vi "Main Target.vi"   [LabVIEW 2018]
uses:
  <vilib>/Platform/TimedLoop/XDataNode/timing_clust.ctl
  <vilib>/Platform/TimedLoop/XDataNode/nitl_modes.ctl
  <vilib>/Platform/TimedLoop/XDataNode/wakeup.ctl
  Host Messages.ctl
  Target Logging Cluster.ctl
  Target Sensors.ctl
  <vilib>/platform/TimedLoop/XDataNode/XDataNode.xnode
  <vilib>/Platform/TimedLoop/XDataNode/XDNodeRunTimeDep.lvlib
types:
  T1 = typedef "XDNodeRunTimeDep.lvlib/timing_clust.ctl" = cluster{"Expected End [f-1]":u64, "Actual End [f-1]":u64, "Finished Late? [f-1]":bool, "Expected End [i-1]":u64, "Actual End [i-1]":u64, "Finished Late? [i-1]":bool, "Expected Start [i]":u64, "Actual Start [i]":u64, "Expected Start [f]":u64, "Actual Start [f]":u64, "Source Name":string, "Structure Name":string, "Period":i64, "Deadline":i64, "Offset":i64, "Start":i64, "Priority":i32, "Timeout":i32, "Mode":T2, "Wakeup Reason":T3, "Error":errorcluster, "Source Type":string, "Secondary Source Type":string, "Global End Time":u64, "Global Start Time":u64, "Frame Duration":u64, "Iteration Duration":u64, "Assigned CPU":i32, "I/O Scan Engine Mode":u32}
  T2 = typedef "XDNodeRunTimeDep.lvlib/nitl_modes.ctl" = enum32{"No Change", "Process missed periods, maintain original phase", "Discard missed periods, maintain original phase", "Process missed periods, ignore original phase", "Discard missed periods, ignore original phase"}
  T3 = typedef "XDNodeRunTimeDep.lvlib/wakeup.ctl" = enum32{"Normal", "Aborted", "Asynchronous wakeup", "Timing source error", "Timed loop error", "Timeout"}
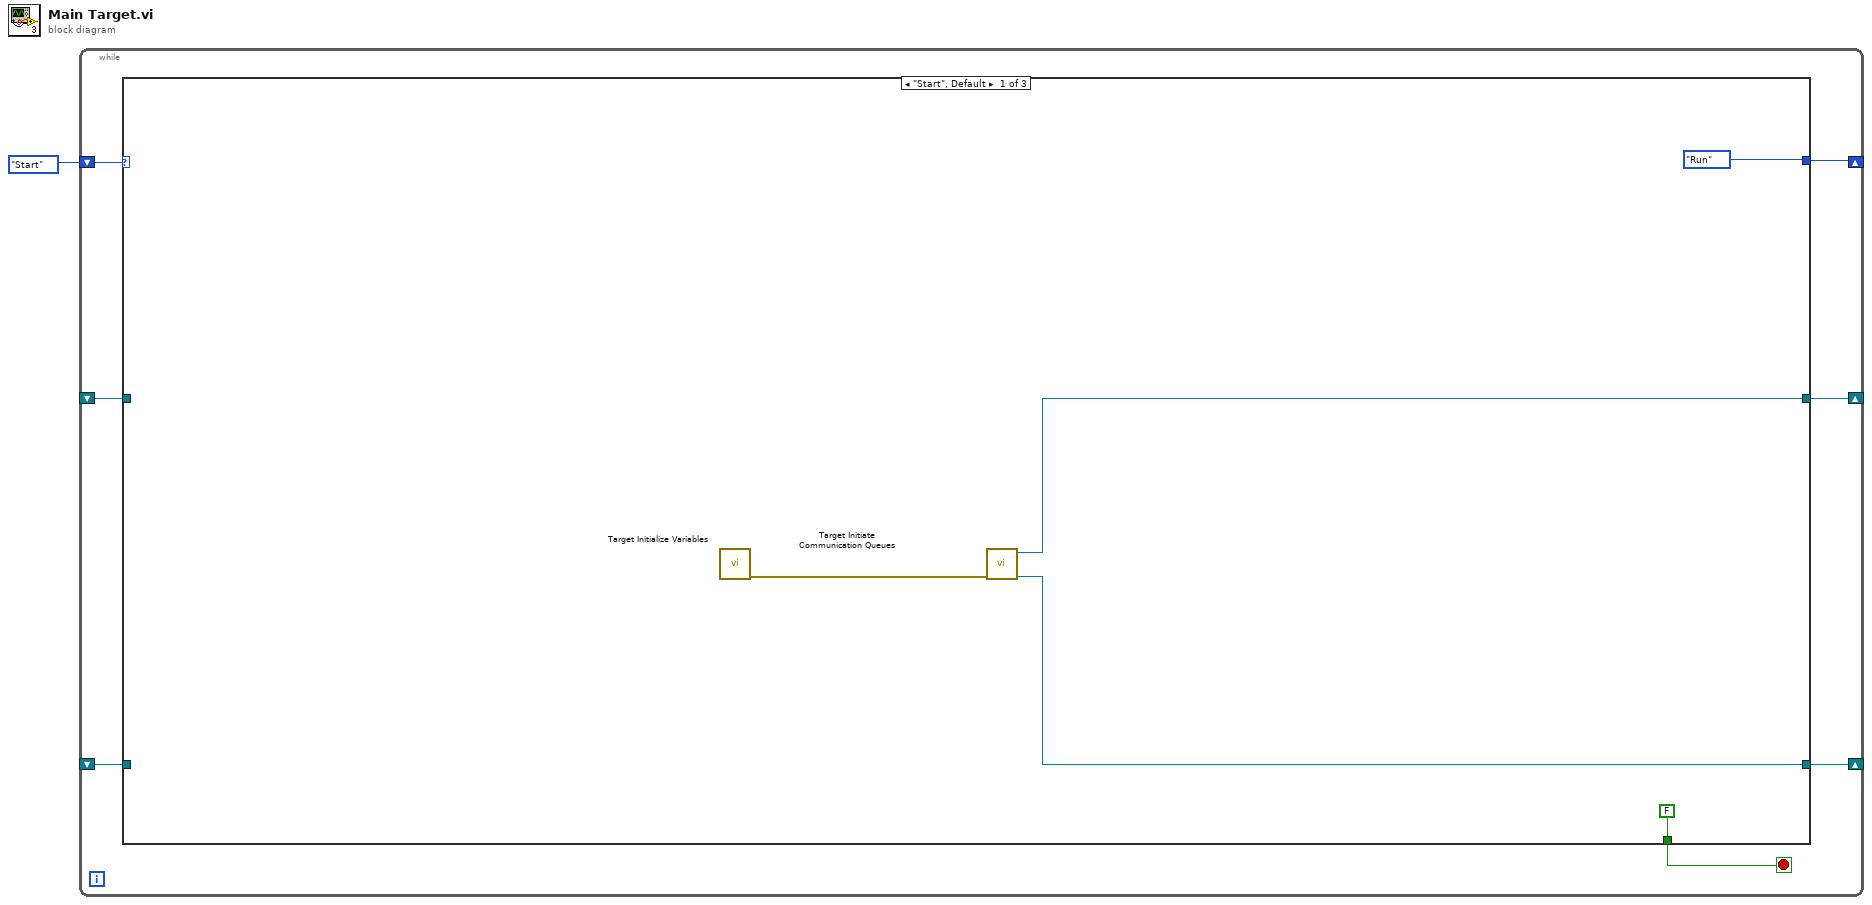
[diagram p0: block diagram]
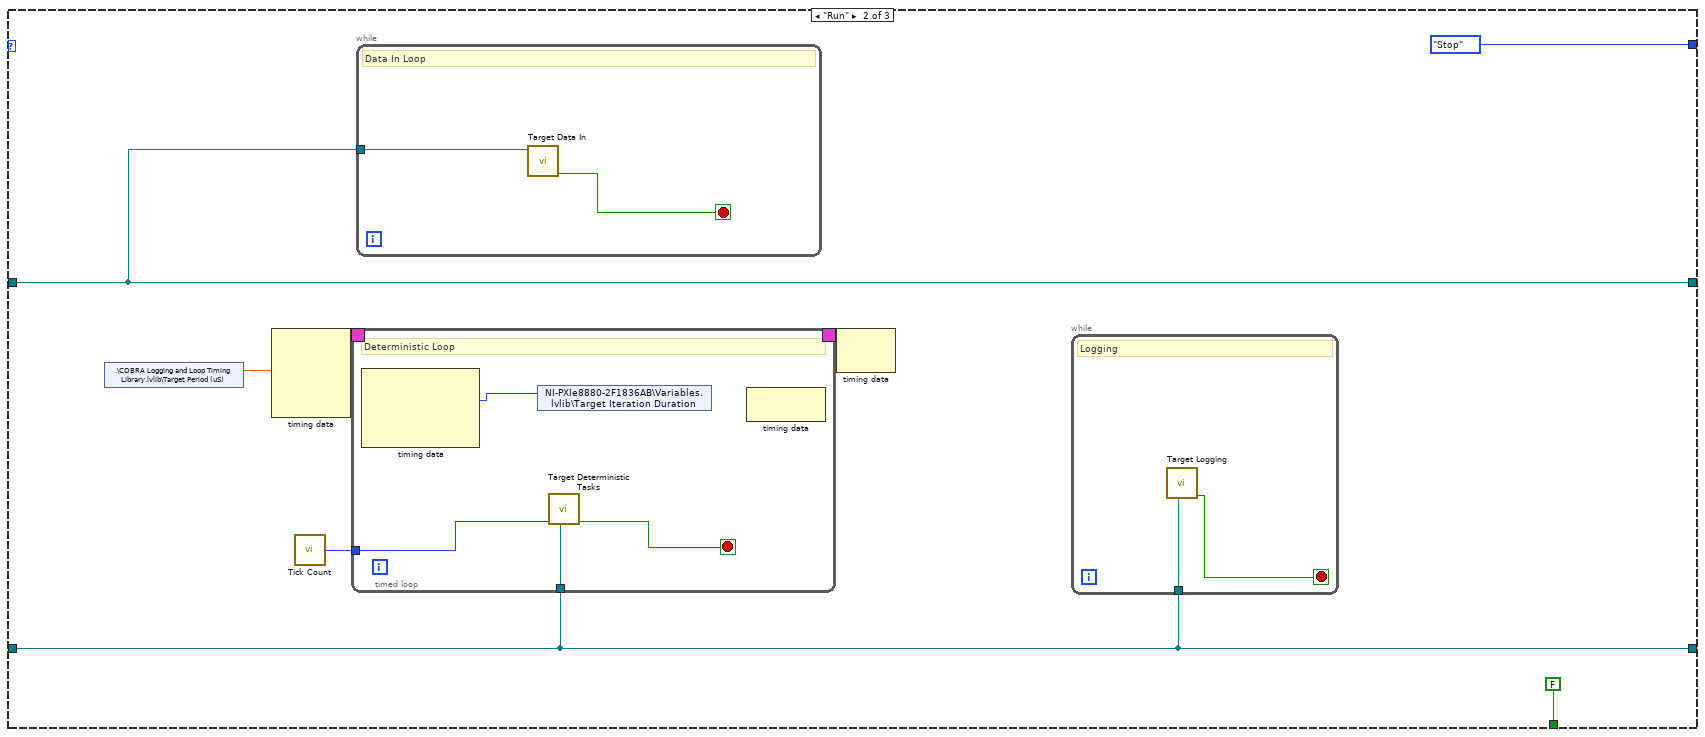
[diagram p2: hidden frame]
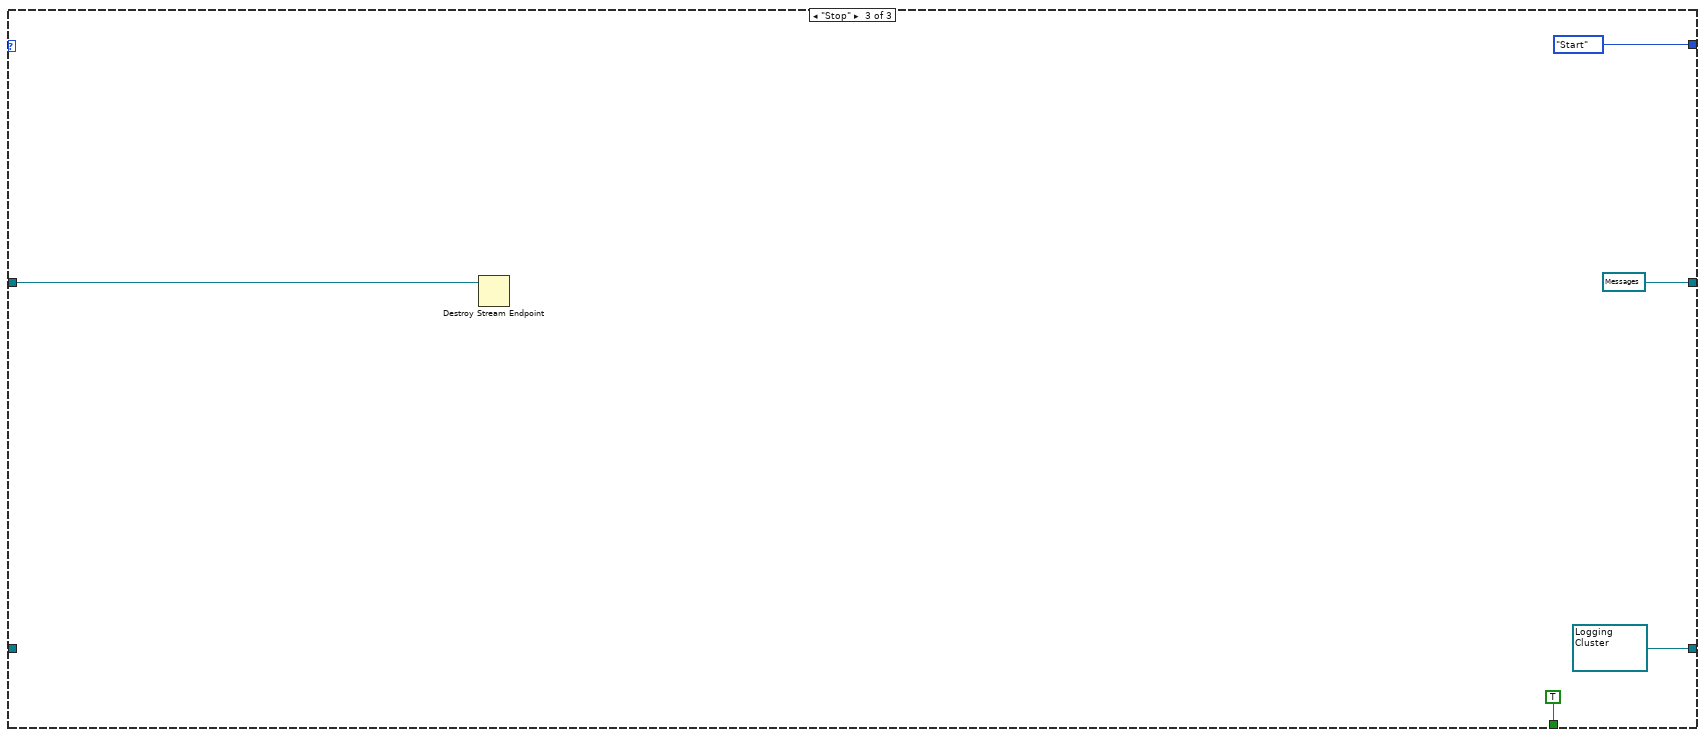
[diagram p3: hidden frame]
diagram:
  n1 = while {
    shift-right: [w7] -> _
    shift-left: enum16{"Start", "Run", "Stop"}."Start" -> [w8]
    shift-right: [w5] -> _
    shift-left: _ -> [w4]
    shift-right: [w3] -> _
    shift-left: _ -> [w2]
    stop <- w6 stop-if-true
    n2 = case shown="\"Start\", Default" w8 {
      tunnel: [enum16{"Start", "Run", "Stop"}."Run" enum16{"Start", "Run", "Stop"}."Stop" enum16{"Start", "Run", "Stop"}."Start"] -> w7
      tunnel: [FALSE FALSE TRUE] -> w6
      tunnel: [w11 w17 w39] -> w5
      tunnel: w4 -> [_ w17 w38]
      tunnel: [w10 w16 refnum<k33> refnum ("rt fifo")] -> w3
      tunnel: w2 -> [_ w16 _]
      frame "Start", Default {
        n3 = call "Target Initialize Variables.vi"() -> ("Error Out"=w9:errorcluster)  [unwired: 11 in]
        n4 = call "Target Initiate Communication Queues.vi"("Error In"=w9) -> ("Refnum out"=w10:refnum<k33>, "writer name"=w11:refnum<k21>)  [unwired: 8 in, 1 out]
      }
      frame "Run" {
        n5 = shared-variable ".\\COBRA Logging and Loop Timing Library.lvlib\\Target Period (uS)"() -> (w14:dbl)  [unwired: 1 in, 1 out]
        n6 = node-c288(w14) -> (w19:T1)  [unwired: 3 in]
        n7 = call "Tick Count"() -> ("Tick Count(uSec)"=w15:u32)
        n8 = timed-loop {
          timing: w19 -> [_]
          timing-out: [_] -> w18
          tunnel: w16 -> [w24]
          tunnel: w15 -> [w23]
          stop <- w25 stop-if-true
          # "Deterministic Loop"
          n9 = node-c288() -> (w22:i64)  [unwired: 1 in, 3 out]
          n10 = shared-variable "NI-PXIe8880-2F1836AB\\Variables.lvlib\\Target Iteration Duration"(w22) -> ()  [unwired: 1 in, 1 out]
          n11 = call "Target Deterministic Tasks.vi"("rt fifo"=w24, "Start Time (uSec)"=w23) -> ("Stop"=w25:bool)  [unwired: 9 in]
          n12 = node-c288() -> ()  [unwired: 1 in, 1 out]
        }
        n13 = while {
          tunnel: w17 -> [w36]
          stop <- w35 stop-if-true
          # "Data In Loop"
          n14 = call "Target Data In.vi"("writer name"=w36) -> ("Stop"=w35:bool)  [unwired: 10 in]
        }
        n15 = node-c288(w18) -> ()  [unwired: 1 out]
        n16 = while {
          tunnel: w16 -> [w34]
          stop <- w33 stop-if-true
          # "Logging"
          n17 = call "Target Logging.vi"("rt fifo"=w34) -> ("Stop Loop"=w33:bool)  [unwired: 10 in]
        }
      }
      frame "Stop" {
        w39 = refnum<k21> refnum items=["Stop", "Log Data", "Confirm File Name"] ("writer name")
        n18 = Destroy Stream Endpoint(11:w38) -> ()  [unwired: 1 in, 1 out]
      }
    }
  }
